vi "Main.vi"() -> ()   [LabVIEW 2017]
doc: "The myRIO Project template acquires acceleration data from the onboard accelerometer and displays the changes of acceleration values in a waveform chart."
uses:
  <vilib>/myRIO/Instrument Drivers/Utilities/Utilities.lvlib
  <vilib>/myRIO/Express VI/Onboard IO/PWM/PWM Express VI.xnode
  <vilib>/myRIO/Instrument Drivers/Onboard IO/PWM/vis/Set Duty Cycle and Frequency.vi
  <vilib>/myRIO/Instrument Drivers/Onboard IO/PWM/PWM.lvlib
  <vilib>/myRIO/Instrument Drivers/Onboard IO/PWM/typedefs/PWM Configuration.ctl
  <vilib>/myRIO/Common/Instrument Driver Framework/myRIO v1.0/PWM/typedefs/PWM Channels Enum.ctl
  <vilib>/myRIO/Common/Instrument Driver Framework/Utilities/typedefs/Generic FPGA Reference.ctl
  <vilib>/myRIO/Common/Instrument Driver Framework/Utilities/typedefs/myRIO v1.0 Reference.ctl
  <vilib>/myRIO/Common/Instrument Driver Framework/Utilities/typedefs/Hardware Version Enum.ctl
  <vilib>/myRIO/Common/Instrument Driver Framework/Utilities/typedefs/myRIO Generic Hardware Reference.ctl
  <vilib>/myRIO/Instrument Drivers/Onboard IO/PWM/typedefs/PWM Reference.ctl
  <vilib>/myRIO/Instrument Drivers/Onboard IO/PWM/vis/myRIO PWM Open.xnode
  <vilib>/myRIO/Common/Instrument Driver Framework/Utilities/vis/Is FPGA Ref Available.vi
  <vilib>/myRIO/Common/Instrument Driver Framework/myRIO v1.0/PWM/vis/myRIO v1.1 Open PWM.vi
  <vilib>/userdefined/High Color/nirio_resource_hc.ctl
  Flow Control Enum.ctl
  Motor Status Enum.ctl
  Motion Type Def.ctl
  XY Cluster.ctl
panel:
  in  "Y Input":T1 {"Tol" min=0.0}
  in  "X Input":T1 {"Tol" min=0.0}
  out "X PID":cluster{"Speed":dbl, "Speed":dbl}(graph)
  out "Next state":T2
  out "State":T2
  out "output cluster":T3
  out "XY Completed?":bool
  in  "Angle Tolerance (°)":dbl=0.5 format="%#_13g"
  out "Kicker Stepper \nON/OFF":bool
  out "Loop Counter":i32
  out "Solenoid\nON/OFF":bool
  out "Kicker Outputs":T4
  out "Y PID":cluster{"Speed":dbl, "Speed":dbl}(graph)
  in  "stop":bool
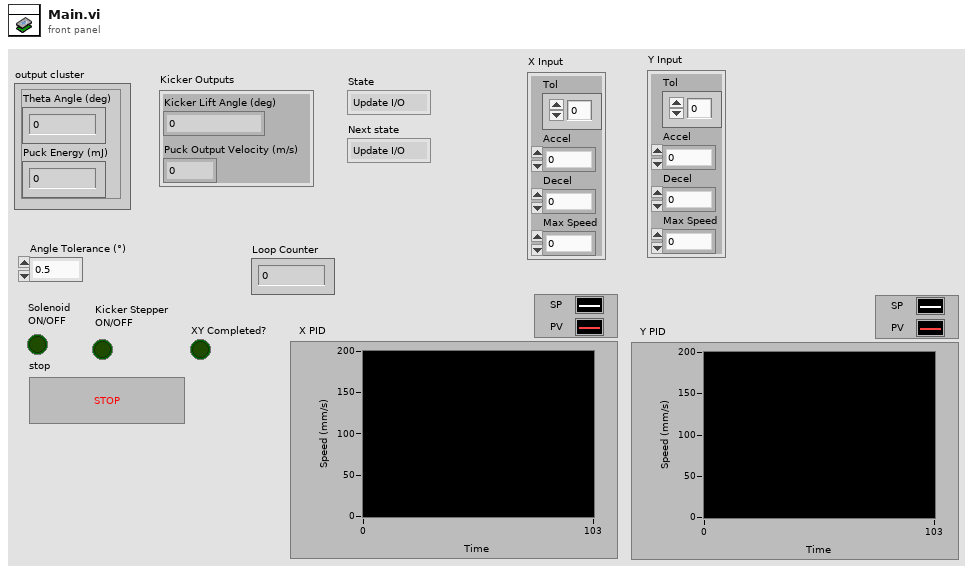
[diagram p1: front panel]
types:
  T1 = cluster{"Tol":dbl, "Accel":dbl, "Decel":dbl, "Max Speed":dbl}
  T2 = typedef "Flow Control Enum.ctl" = enum16{"Update I/O", "Kicker", "XY Drive", "Theta Axis", "Solenoid"}
  T3 = cluster{"Theta Angle (deg)":dbl, "Puck Energy (mJ)":dbl}
  T4 = cluster{"Kicker Lift Angle (deg)":dbl, "Puck Output Velocity (m/s)":dbl}
  T5 = typedef "XY Cluster.ctl" = cluster{"X Data":cluster{"Complete?":bool, "Motor Params":cluster{"Duty %":dbl, "X Freq":dbl, "FWD/RVS":bool}, "SP":cluster{"Accel":dbl, "Decel":dbl, "Speed":dbl}, "State":T6, "Input":cluster{"Coord":dbl, "Tol":dbl, "Accel":dbl, "Decel":dbl, "Max Speed":dbl}, "Path":cluster{"V plan":dbl[], "V actual":dbl[], "S actual":dbl[], "a actual":dbl[], "Profile":T7, "Decel Dist":dbl, "Accel Dist":dbl, "Cruise V":dbl, "Cruise Dist":dbl}, "PID":cluster{"Kc":dbl, "Ti":dbl, "Td":dbl}, "Motion":cluster{"Speed":dbl, "Dist":dbl, "Acceleration":dbl, "Dist to target":dbl}}, "Y Data":cluster{"Complete?":bool, "Motor Params":cluster{"Duty %":dbl, "Freq":dbl, "FWD/RVS":bool}, "SP":cluster{"Y Accel":dbl, "Y Decel":dbl, "Speed":dbl}, "State":T6, "Input":cluster{"Coord":dbl, "Tol":dbl, "Accel":dbl, "Decel":dbl, "Max Speed":dbl}, "Path":cluster{"V plan":dbl[], "V actual":dbl[], "S actual":dbl[], "a actual":dbl[], " Profile":T7, "Decel Dist":dbl, "Accel Dist":dbl, "Cruise V":dbl, "Cruise Dist":dbl}, "PID":cluster{"Kc":dbl, "Ti":dbl, "Td":dbl}, "Motion":cluster{"Speed":dbl, "Dist":dbl, "Acceleration":dbl, "Dist to target":dbl}}, "Timing":cluster{"Runtime":dbl, "Loop time":dbl, "Loop iter":i32, "Tick":dbl}, "stop":bool}
  T6 = typedef "Motor Status Enum.ctl" = enum16{"Update I/O", "Stop", "Steady Speed", "Accelerate", "Decelerate", "Drive Motor"}
  T7 = typedef "Motion Type Def.ctl" = enum16{"Trapezodial", "Triangular"}
  T8 = cluster{"Kicker Inputs":cluster{"Theta Angle (deg)":dbl, "Puck Energy (mJ)":dbl}, "Kicker Outputs":cluster{"Kicker Lift Angle (deg)":dbl, "Puck Output Velocity (m/s)":dbl}, "Solenoid\nON/OFF":bool, "Kicker Stepper \nON/OFF":bool, "Angle Tolerance (°)":dbl, "Current Motor Step":i32}
  T9 = cluster{"Kicked?":bool, "Stop?":bool, "State":T2}
  T10 = cluster{"X Coord":dbl, "Y Coord":dbl, "Energy":dbl, "Theta Angle":dbl}
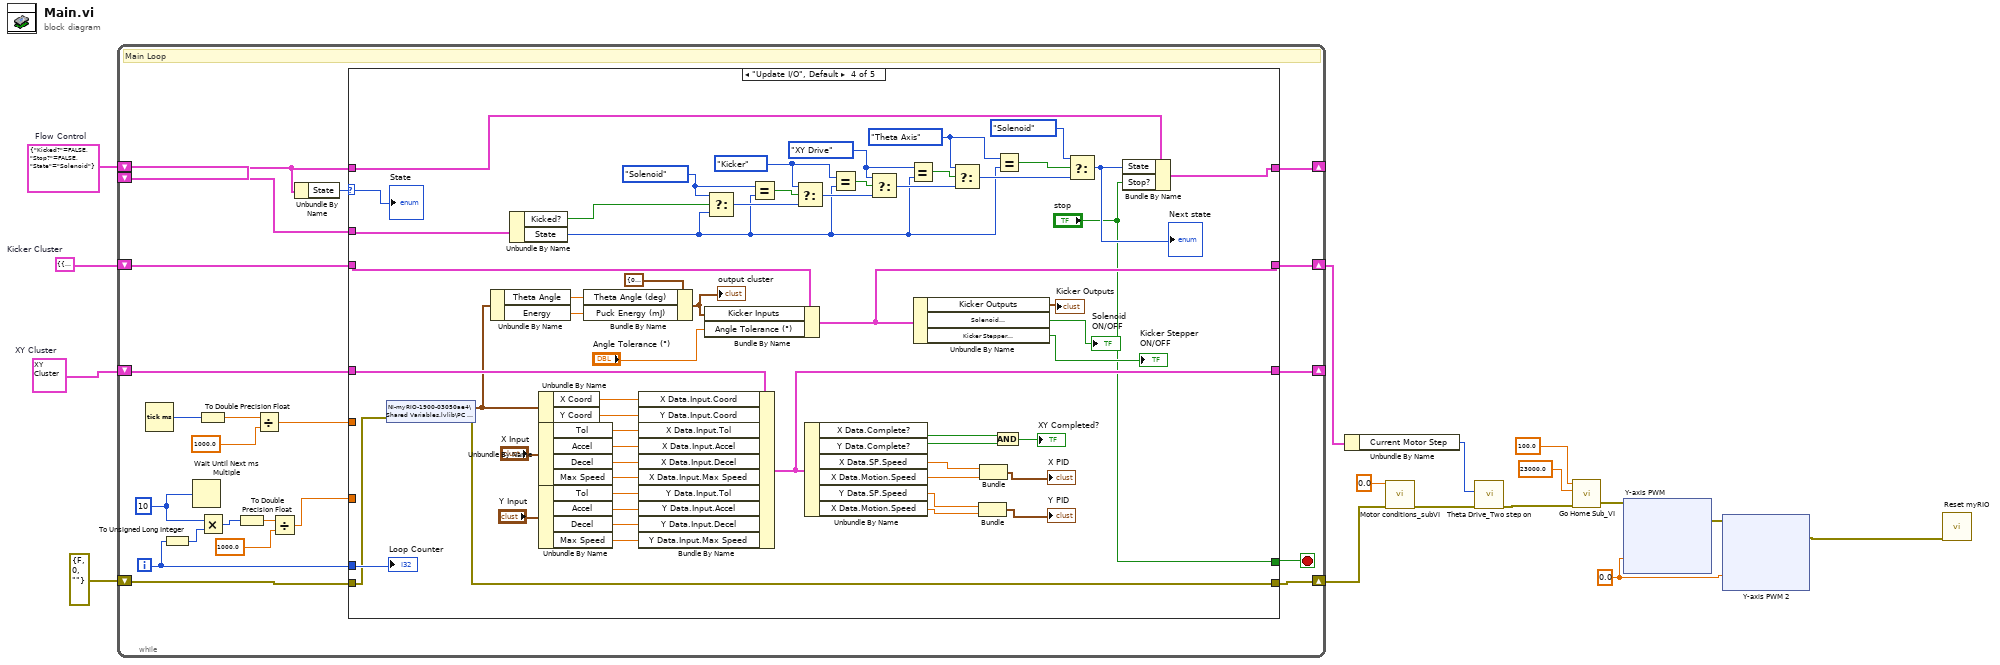
[diagram p0: block diagram]
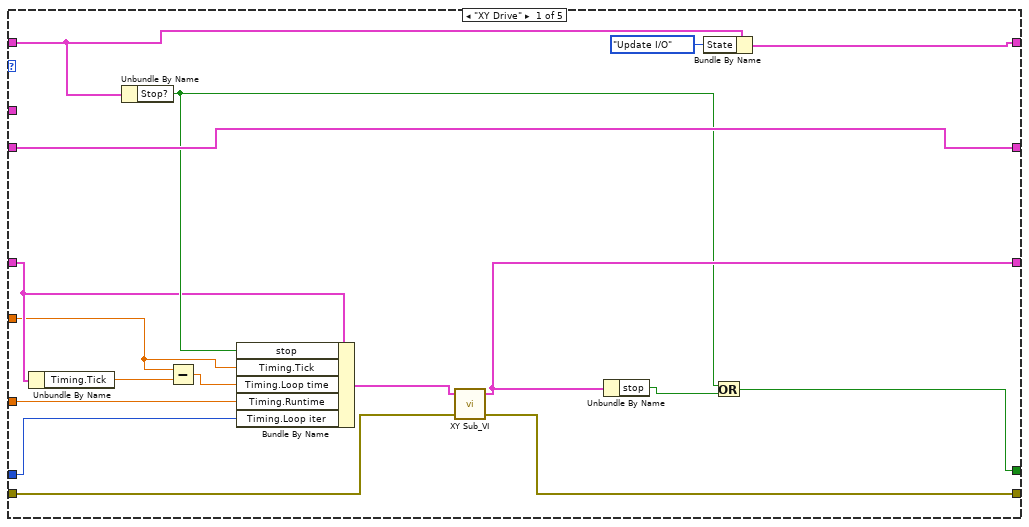
[diagram p2: hidden frame]
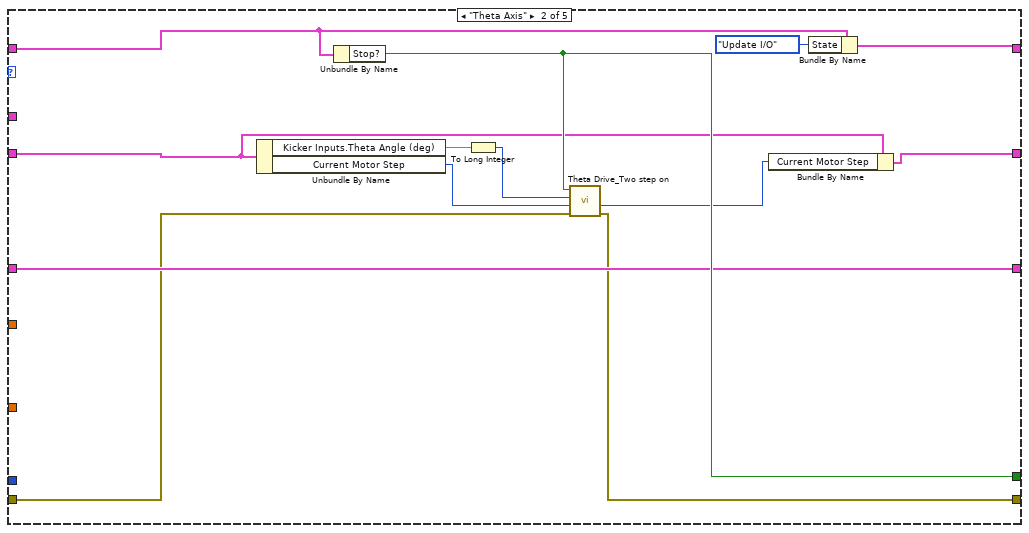
[diagram p3: hidden frame]
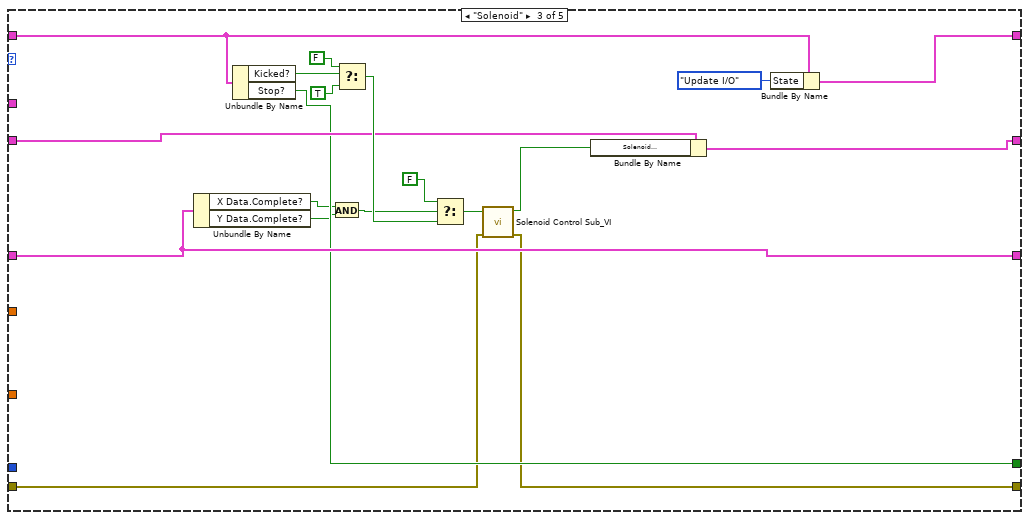
[diagram p4: hidden frame]
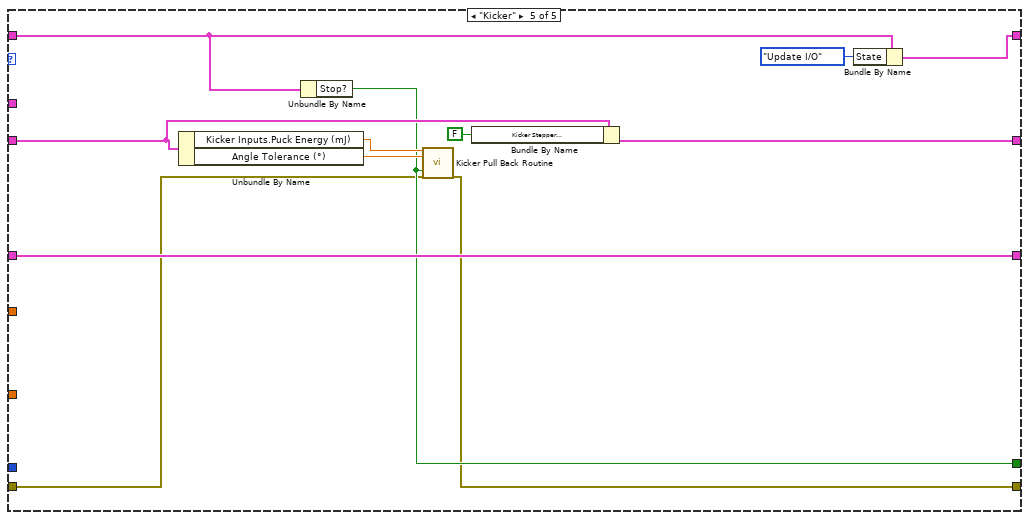
[diagram p5: hidden frame]
diagram:
  w2 = T5 {"X Data"={"Complete?"=FALSE, "Motor Params"={"Duty %"=0.0, "X Freq"=0.0, "FWD/RVS"=FALSE}, "SP"={"Accel"=0.0, "Decel"=0.0, "Speed"=0.0}, "State"=enum."Update I/O", "Input"={"Coord"=0.0, "Tol"=0.0, "Accel"=0.0, "Decel"=0.0, "Max Speed"=0.0}, "Path"={"V plan"=[], "V actual"=[], "S actual"=[], "a actual"=[], "Profile"=enum."Trapezodial", "Decel Dist"=0.0, "Accel Dist"=0.0, "Cruise V"=0.0, "Cruise Dist"=0.0}, "PID"={"Kc"=0.0, "Ti"=0.0, "Td"=0.0}, "Motion"={"Speed"=0.0, "Dist"=0.0, "Acceleration"=0.0, "Dist to target"=0.0}}, "Y Data"={"Complete?"=FALSE, "Motor Params"={"Duty %"=0.0, "Freq"=0.0, "FWD/RVS"=FALSE}, "SP"={"Y Accel"=0.0, "Y Decel"=0.0, "Speed"=0.0}, "State"=enum."Update I/O", "Input"={"Coord"=0.0, "Tol"=0.0, "Accel"=0.0, "Decel"=0.0, "Max Speed"=0.0}, "Path"={"V plan"=[], "V actual"=[], "S actual"=[], "a actual"=[], " Profile"=enum."Trapezodial", "Decel Dist"=0.0, "Accel Dist"=0.0, "Cruise V"=0.0, "Cruise Dist"=0.0}, "PID"={"Kc"=0.0, "Ti"=0.0, "Td"=0.0}, "Motion"={"Speed"=0.0, "Dist"=0.0, "Acceleration"=0.0, "Dist to target"=0.0}}, "Timing"={"Runtime"=0.0, "Loop time"=0.0, "Loop iter"=0, "Tick"=0.0}, "stop"=FALSE}  # XY Cluster
  w3 = T8 {"Kicker Inputs"={"Theta Angle (deg)"=0.0, "Puck Energy (mJ)"=0.0}, "Kicker Outputs"={"Kicker Lift Angle (deg)"=0.0, "Puck Output Velocity (m/s)"=0.0}, "Solenoid\nON/OFF"=FALSE, "Kicker Stepper \nON/OFF"=FALSE, "Angle Tolerance (°)"=0.5, "Current Motor Step"=0}  # Kicker Cluster
  w4 = T9 {"Kicked?"=FALSE, "Stop?"=FALSE, "State"=enum."Solenoid"}  # Flow Control
  w14 = 0.0 ("Frequency [Hz]")
  n1 = while {
    shift-right: [w30] -> w11
    shift-left: errorcluster {"status"=FALSE, "code"=0, "source"=""} ("error in (no error)") -> [w31]
    shift-right: [w35] -> _
    shift-left: w4 -> [w38]
    shift-right: [w32] -> _
    shift-left: w2 -> [w25]
    shift-right: [w33] -> w5
    shift-left: w3 -> [w34]
    shift-left: w4 -> [w29]
    i -> [w18]
    stop <- w36 stop-if-true
    w23 = u32 10 ("millisecond multiple")
    # "Main Loop"
    n2 = Tick Count (ms)() -> (millisecond timer value=w28:u32)
    n3 = To Unsigned Long Integer(number=w18) -> (unsigned 32bit integer=w22:u32)
    n4 = Wait Until Next ms Multiple(millisecond multiple=w23) -> ()  [unwired: 1 out]
    n5 = To Double Precision Float(number=w28) -> (double precision float=w26:dbl)
    n6 = Multiply(x=w23, y=w22) -> (x*y=w21:u32)
    n7 = To Double Precision Float(number=w21) -> (double precision float=w19:dbl)
    n8 = Divide(x=w26, y=1000.0) -> (x/y=w24:dbl)
    n9 = Divide(x=w19, y=1000.0) -> (x/y=w17:dbl)
    n10 = Unbundle By Name(w38) -> ("State"=w37:T2)
    n11 = case shown="\"Update I/O\", Default" w37 {
      selector: w37 -> [_ _ _ w109 _]
      tunnel: w38 -> [w52 w66 w77 w123 w151]
      tunnel: [w48 w65 w74 "stop" w149] -> w36
      tunnel: [w54 w67 w76 w122 w157] -> w35
      tunnel: w18 -> [w44 _ _ w145 _]
      tunnel: w25 -> [w43 w58 w78 w138 w150]
      tunnel: w34 -> [w53 w61 w81 w140 w153]
      tunnel: [w53 w60 w80 w139 w152] -> w33
      tunnel: [w47 w58 w78 w137 w150] -> w32
      tunnel: w31 -> [w51 w57 w73 w111 w148]
      tunnel: [w50 w56 w72 w110 w147] -> w30
      tunnel: w29 -> [_ _ _ w119 _]
      tunnel: w24 -> [w40 _ _ _ _]
      tunnel: w17 -> [w39 _ _ _ _]
      frame "XY Drive" {
        n12 = Unbundle By Name(w43) -> ("Timing.Tick"=w42:dbl)
        n13 = Unbundle By Name(w52) -> ("Stop?"=w45:bool)
        n14 = Subtract(x=w40, y=w42) -> (x-y=w41:dbl)
        n15 = Bundle By Name(cluster=w43, "stop"=w45, "Timing.Tick"=w40, "Timing.Loop time"=w41, "Timing.Runtime"=w39, "Timing.Loop iter"=w44) -> (w49:T5)
        n16 = call "XY Sub_VI.vi"("error in (no error)"=w51, "XY Cluster In"=w49) -> ("error out"=w50:errorcluster, "XY Cluster Out"=w47:T5)  [unwired: 2 in]
        n17 = Unbundle By Name(w47) -> ("stop"=w46:bool)
        n18 = Bundle By Name(cluster=w52, "State"=Flow_Control_Enum."Update I/O") -> (w54:T9)
        n19 = Or(x=w45, y=w46) -> (x .or. y?=w48:bool)
      }
      frame "Theta Axis" {
        n20 = Unbundle By Name(w61) -> ("Kicker Inputs.Theta Angle (deg)"=w64:dbl, "Current Motor Step"=w62:i32)
        n21 = Unbundle By Name(w66) -> ("Stop?"=w65:bool)
        n22 = To Long Integer(number=w64) -> (32bit integer=w63:i32)
        n23 = call "Theta Drive_Two step on.vi"("error in (no error)"=w57, "Start Location Step (-90to90)"=w62, "Target Step (-90to90)"=w63, "stop"=w65) -> ("error out"=w56:errorcluster, "Current Motor Step (0to3)"=w59:i32)  [unwired: 4 in, 2 out]
        n24 = Bundle By Name(cluster=w61, "Current Motor Step"=w59) -> (w60:T8)
        n25 = Bundle By Name(cluster=w66, "State"=Flow_Control_Enum."Update I/O") -> (w67:T9)
      }
      frame "Solenoid" {
        n26 = Unbundle By Name(w78) -> ("X Data.Complete?"=w71:bool, "Y Data.Complete?"=w70:bool)
        n27 = Unbundle By Name(w77) -> ("Kicked?"=w87:bool, "Stop?"=w74:bool)
        n28 = And(x=w71, y=w70) -> (x .and. y?=w69:bool)
        n29 = Select(t=FALSE, s=w87, f=TRUE) -> (s? t:f=w83:bool)
        n30 = Select(t=FALSE, s=w69, f=w83) -> (s? t:f=w82:bool)
        n31 = call "Solenoid Control Sub_VI.vi"("error in (no error)"=w73, "SOLENOID ON/OFF"=w82) -> ("error out"=w72:errorcluster, "ON/OFF"=w79:bool)  [unwired: 8 in]
        n32 = Bundle By Name(cluster=w81, "Solenoid\nON/OFF"=w79) -> (w80:T8)
        n33 = Bundle By Name(cluster=w77, "State"=Flow_Control_Enum."Update I/O") -> (w76:T9)
      }
      frame "Update I/O", Default {
        w129 = Flow_Control_Enum."Theta Axis" ("State")
        w132 = Flow_Control_Enum."XY Drive" ("State")
        w133 = Flow_Control_Enum."Kicker" ("State")
        w134 = Flow_Control_Enum."Solenoid" ("State")
        n34 = shared-variable "NI-myRIO-1900-03050ae4\\Shared Variables.lvlib\\PC To Rio"(error in=w111) -> (w114:T10, error out=w110:errorcluster)
        n35 = Unbundle By Name(w114) -> ("Theta Angle"=w112:dbl, "Energy"=w113:dbl)
        n36 = Unbundle By Name(w119) -> ("Kicked?"=w118:bool, "State"=w117:T2)
        n37 = Unbundle By Name(w114) -> ("X Coord"=w108:dbl, "Y Coord"=w107:dbl)
        n38 = Unbundle By Name("X Input") -> ("Tol"=w96:dbl, "Accel"=w95:dbl, "Decel"=w94:dbl, "Max Speed"=w93:dbl)
        n39 = Unbundle By Name("Y Input") -> ("Tol"=w91:dbl, "Accel"=w90:dbl, "Decel"=w89:dbl, "Max Speed"=w88:dbl)
        n40 = Bundle By Name(cluster=T3 {"Theta Angle (deg)"=0.0, "Puck Energy (mJ)"=0.0} ("Kicker Inputs"), "Theta Angle (deg)"=w112, "Puck Energy (mJ)"=w113) -> (w116:T3)
        "output cluster" <- w116
        n41 = Bundle By Name(cluster=w138, "X Data.Input.Coord"=w108, "Y Data.Input.Coord"=w107, "X Data.Input.Tol"=w96, "X Data.Input.Accel"=w95, "X Data.Input.Decel"=w94, "X Data.Input.Max Speed"=w93, "Y Data.Input.Tol"=w91, "Y Data.Input.Accel"=w90, "Y Data.Input.Decel"=w89, "Y Data.Input.Max Speed"=w88) -> (w137:T5)
        n42 = Bundle By Name(cluster=w140, "Kicker Inputs"=w116, "Angle Tolerance (°)"="Angle Tolerance (°)") -> (w139:T8)
        n43 = Select(t=w134, s=w118, f=w117) -> (s? t:f=w135:T2)
        n44 = Equal?(x=w134, y=w117) -> (x = y?=w136:bool)
        n45 = Select(t=w133, s=w136, f=w135) -> (s? t:f=w130:T2)
        n46 = Unbundle By Name(w137) -> ("X Data.Complete?"=w106:bool, "Y Data.Complete?"=w105:bool, "X Data.SP.Speed"=w102:dbl, "X Data.Motion.Speed"=w101:dbl, "Y Data.SP.Speed"=w99:dbl, "X Data.Motion.Speed"=w98:dbl)
        n47 = Equal?(x=w133, y=w117) -> (x = y?=w131:bool)
        n48 = Select(t=w132, s=w131, f=w130) -> (s? t:f=w127:T2)
        n49 = Equal?(x=w132, y=w117) -> (x = y?=w128:bool)
        n50 = Unbundle By Name(w139) -> ("Kicker Outputs"=→"Kicker Outputs":T4, "Solenoid\nON/OFF"=→"Solenoid\nON/OFF":bool, "Kicker Stepper \nON/OFF"=→"Kicker Stepper \nON/OFF":bool)
        n51 = Select(t=w129, s=w128, f=w127) -> (s? t:f=w124:T2)
        n52 = Bundle("Speed"=w99, "Speed"=w98) -> (→"Y PID":cluster{"Speed":dbl, "Speed":dbl})  [unwired: 1 in]
        n53 = Bundle("Speed"=w102, "Speed"=w101) -> (→"X PID":cluster{"Speed":dbl, "Speed":dbl})  [unwired: 1 in]
        n54 = And(x=w106, y=w105) -> (x .and. y?=→"XY Completed?":bool)
        n55 = Equal?(x=w129, y=w117) -> (x = y?=w125:bool)
        n56 = Select(t=Flow_Control_Enum."Solenoid" ("State"), s=w125, f=w124) -> (s? t:f=w121:T2)
        "Next state" <- w121
        n57 = Bundle By Name(cluster=w123, "State"=w121, "Stop?"="stop") -> (w122:T9)
        "Loop Counter" <- w145
        "State" <- w109
      }
      frame "Kicker" {
        n58 = Unbundle By Name(w153) -> ("Kicker Inputs.Puck Energy (mJ)"=w155:dbl, "Angle Tolerance (°)"=w154:dbl)
        n59 = Unbundle By Name(w151) -> ("Stop?"=w149:bool)
        n60 = call "Kicker Pull Back Routine.vi"("Puck Energy Requirement (mJ)"=w155, "Angle Tolerance (°)"=w154, "stop"=w149, "error in (no error)"=w148) -> ("error out"=w147:errorcluster)  [unwired: 13 in, 2 out]
        n61 = Bundle By Name(cluster=w153, "Kicker Stepper \nON/OFF"=FALSE ("Kicker Stepper \nON/OFF")) -> (w152:T8)
        n62 = Bundle By Name(cluster=w151, "State"=Flow_Control_Enum."Update I/O") -> (w157:T9)
      }
    }
  }
  n63 = Unbundle By Name(w5) -> ("Current Motor Step"=w6:i32)
  n64 = call "Motor conditions_subVI.vi"("Target Angle (°)"=0.0, "error in (no error)"=w11) -> ("error out"=w10:errorcluster)  [unwired: 11 in, 2 out]
  n65 = call "Theta Drive_Two step on.vi"("error in (no error)"=w10, "Target Step (-90to90)"=w6) -> ("error out"=w9:errorcluster)  [unwired: 6 in, 3 out]
  n66 = call "Go Home Sub_VI.vi"("error in (no error)"=w9, "Homing Freq"=23000.0, "Homing Duty %"=100.0) -> ("error out"=w7:errorcluster)  [unwired: 7 in, 1 out]
  n67 = xnode "Y-axis PWM"("Frequency [Hz]"=w14, "error in (no error)"=w7) -> ("error out"=w15:errorcluster)
  n68 = xnode "Y-axis PWM 2"("Frequency [Hz]"=w14, "error in (no error)"=w15) -> ("error out"=w1:errorcluster)
  n69 = call <vilib>:"Reset myRIO.vi"("error in (no error)"=w1) -> ()  [unwired: 10 in, 1 out]
